vi "Count_Triggers.vi"(9 "Max Triggers":i32, 10 "Triggers In":u64, 11 "channel":u32) -> (1 "Coincidence Triggers":u64, 2 "Max triggers?":bool, 3 "Total Triggers Out":u64)   [LabVIEW 2023]
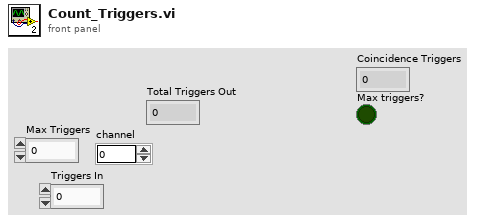
[diagram p1: front panel]
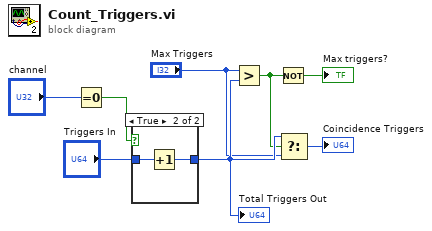
[diagram p0: block diagram]
diagram:
  n1 = Equal To 0?(x="channel") -> (x = 0?=w8:bool)
  n2 = case shown="True" w8 {
    tunnel: "Triggers In" -> [w9 w11]
    tunnel: [w9 w10] -> w6
    frame False {
    }
    frame True {
      n3 = Increment(x=w11) -> (x+1=w10:u64)
    }
  }
  "Total Triggers Out" <- w6
  n4 = Greater?(x="Max Triggers", y=w6) -> (0:w2:bool)
  n5 = Not(x=w2) -> (.not. x?=→"Max triggers?":bool)
  n6 = Select(t=w6, s=w2, f="Max Triggers") -> (s? t:f=→"Coincidence Triggers":u64)
